vi "Actor Core.vi"(8 "error in":errorcluster, 11 "Controller in":refnum<class "Controller.lvclass">) -> (0 "error out":errorcluster, 3 "Actor out":refnum<class "Actor.lvclass">)   [LabVIEW 2020, in "Controller.lvlib" / "Controller.lvclass"]
doc: "(<B>Filename</B>: Actor Framework.lvlib:Actor.lvclass:Actor Core.vi)\n\nReceives messages to the actor, reacts to them, and initiates any error handling that may shut the actor down.\n\nDescendant classes may override this VI to append parallel tasks for the actor to complete while it handles messages. Overrides use the Call Parent Class Method node."
uses:
  Controller.lvclass
  C:/Program Files/National Instruments/LabVIEW 2020/vi.lib/ActorFramework/Actor/Actor.lvclass
  <vilib>/ActorFramework/Actor/Actor.lvclass
  Main_UI/Main_UI/Main_UI.lvclass
  Actor_log/Actor_log/Actor_log.lvclass
  Actor_NI6008/Actor_NI6008/Actor_NI6008.lvclass
  Controller.lvclass/Controller.ctl
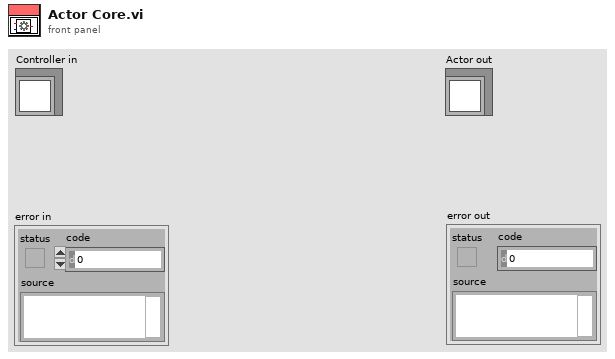
[diagram p1: front panel]
types:
  T1 = enum16{"open", "replace", "create", "open or create", "replace or create", "replace or create with confirmation"}
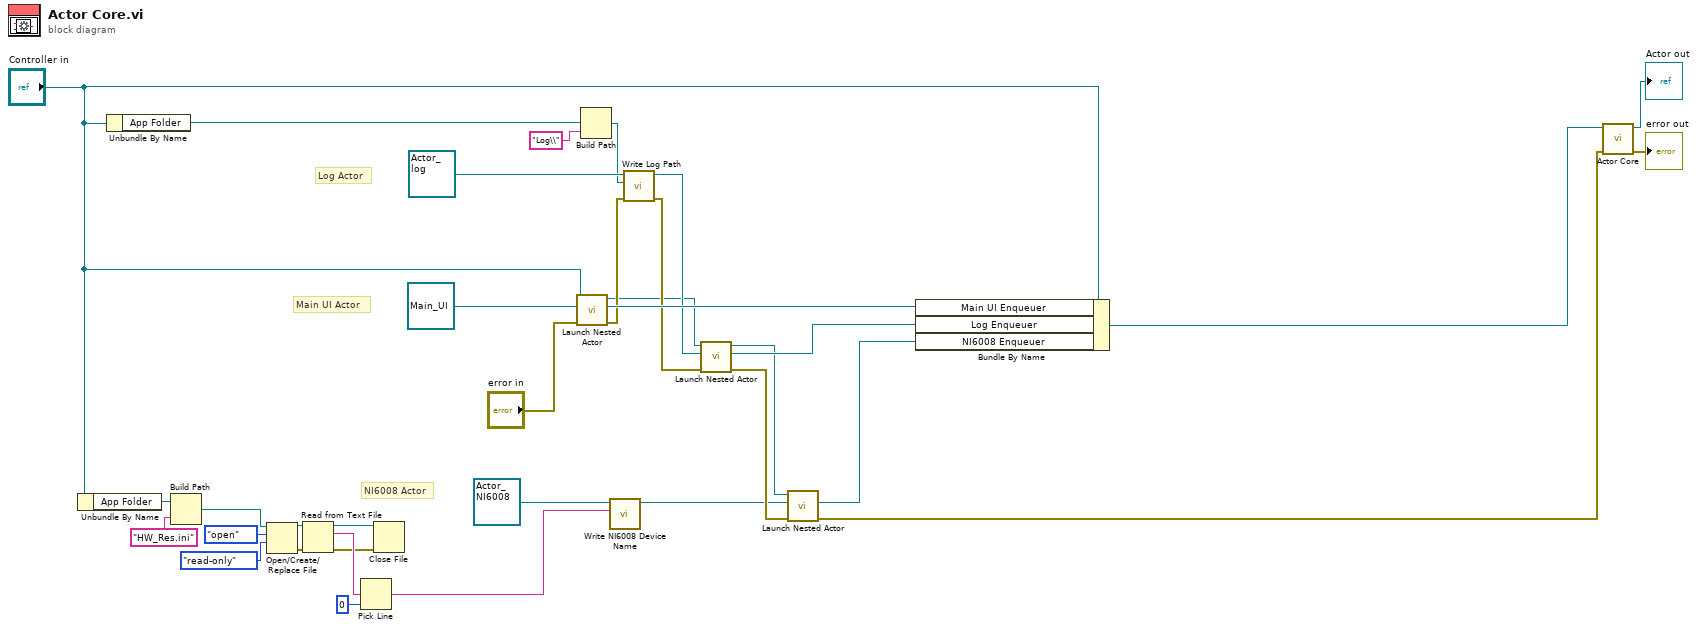
[diagram p0: block diagram]
diagram:
  # "NI6008 Actor"
  # "Log Actor"
  # "Main UI Actor"
  n1 = Unbundle By Name("Controller in") -> ("App Folder"=w4:path)
  n2 = Unbundle By Name("Controller in") -> ("App Folder"=w28:path)
  n3 = Build Path(base path=w4, name or relative path="HW_Res.ini") -> (appended path=w9:path)
  n4 = Open/Create/Replace File(file path (use dialog)=w9, operation (0:open)=T1."open", access (0:read/write)=enum16{"read/write", "read-only", "write-only"}."read-only") -> (refnum out=w8:refnum<file>, error out=w7:errorcluster)  [unwired: 3 in, 1 out]
  n5 = Read from Text File(file (use dialog)=w8, error in=w7) -> (refnum out=w1:refnum<file>, text=w5:string, error out=w2:errorcluster)  [unwired: 2 in, 1 out]
  n6 = Pick Line(multi-line string=w5, line index=0) -> (output string=w3:string)  [unwired: 1 in]
  n7 = Close File(refnum=w1, error in=w2) -> ()  [unwired: 2 out]
  n8 = call <vilib>:"Launch Nested Actor.vi"("error in (no error)"="error in", "Nested Actor"=refnum<class "Main_UI.lvclass"> refnum ("Main_UI.lvlib:Main_UI.lvclass"), "Caller Actor in"="Controller in") -> ("error out"=w24:errorcluster, "Nested Actor's Enqueuer"=w32:refnum<class "Message Enqueuer.lvclass">, "Caller Actor out"=w21:refnum<class "Controller.lvclass">)  [unwired: 6 in]
  n9 = Build Path(base path=w28, name or relative path="Log\\") -> (appended path=w25:path)
  n10 = call-dynamic "Write NI6008 Device Name.vi"("NI6008 Device Name"=w3, "Actor_NI6008 in"=refnum<class "Actor_NI6008.lvclass"> refnum ("Actor_NI6008.lvlib:Actor_NI6008.lvclass")) -> ("Actor_NI6008 out"=w14:refnum<class "Actor_NI6008.lvclass">)  [unwired: 8 in, 1 out]
  n11 = call-dynamic "Write Log Path.vi"("error in (no error)"=w24, "Log Path"=w25, "Actor_log in"=refnum<class "Actor_log.lvclass"> refnum ("Actor_log.lvlib:Actor_log.lvclass")) -> ("error out"=w23:errorcluster, "Actor_log out"=w22:refnum<class "Actor_log.lvclass">)  [unwired: 7 in]
  n12 = call <vilib>:"Launch Nested Actor.vi"("error in (no error)"=w23, "Nested Actor"=w22, "Caller Actor in"=w21) -> ("error out"=w17:errorcluster, "Nested Actor's Enqueuer"=w20:refnum<class "Message Enqueuer.lvclass">, "Caller Actor out"=w19:refnum<class "Controller.lvclass">)  [unwired: 6 in]
  n13 = call <vilib>:"Launch Nested Actor.vi"("error in (no error)"=w17, "Nested Actor"=w14, "Caller Actor in"=w19) -> ("error out"=w16:errorcluster, "Nested Actor's Enqueuer"=w18:refnum<class "Message Enqueuer.lvclass">)  [unwired: 6 in, 1 out]
  n14 = Bundle By Name(cluster="Controller in", "Main UI Enqueuer"=w32, "Log Enqueuer"=w20, "NI6008 Enqueuer"=w18) -> (w29:refnum<class "Controller.lvclass">)
  n15 = call-parent "Actor Core.vi"("error in"=w16, "Actor in"=w29) -> ("error out"=→"error out":errorcluster, "Actor out"=→"Actor out":refnum<class "Actor.lvclass">)  [unwired: 8 in]
